vi "7L19-c-stockage_oui_non.vi"(5 "err in":errorcluster, 8 "Pénalité (e)":T2, 9 "Pièce (e)":T1) -> (1 "Stockage (sortie)":T3, 2 "Pénalité (s)":T2, 3 "Pièce (s)":T1, 4 "err out":errorcluster)   [LabVIEW 2010, in "lv_07.lvlib"]
doc: "Evalue dans la commande Stockage si la pièce peut être stockée - \n- Valeur de Qa min à comparer à Qa\n- CDM > CSM ?"
uses:
  lv_07.lvlib
  c_pi_wilson.ctl
  c_pi_penalite.ctl
  c_pi_stock.ctl
  c_pi_stock_O-N.ctl
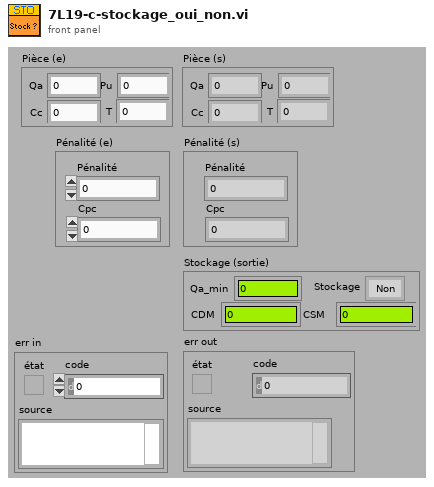
[diagram p1: front panel]
types:
  T1 = typedef "lv_07.lvlib/c_pi_wilson.ctl" = cluster{"T":dbl, "Pu":dbl, "Qa":dbl, "Cc":dbl}
  T2 = typedef "lv_07.lvlib/c_pi_penalite.ctl" = cluster{"Pénalité":dbl, "Cpc":dbl}
  T3 = typedef "lv_07.lvlib/c_pi_stock.ctl" = cluster{"Qa_min":dbl, "CDM":dbl, "CSM":dbl, "Stockage":T4}
  T4 = typedef "lv_07.lvlib/c_pi_stock_O-N.ctl" = enum16{"Non", "Oui"}
  T5 = typedef "lv_07.lvlib/c_cout_choix_q.ctl" = cluster{"Cadm":dbl, "Cpos":dbl, "Cach":dbl, "CSM":dbl, "q":dbl, "T en mois":dbl}
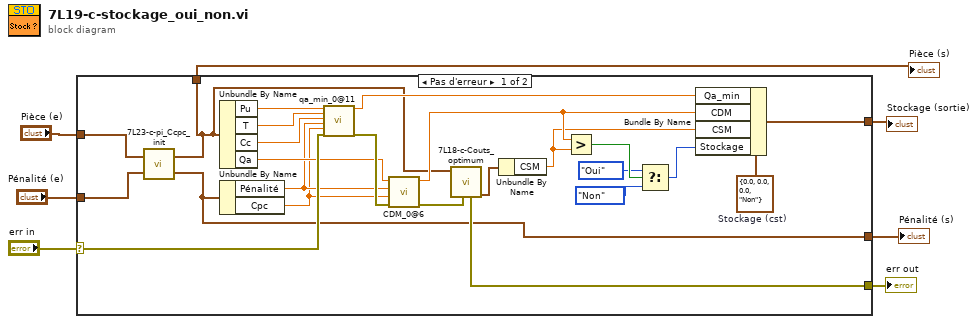
[diagram p0: block diagram]
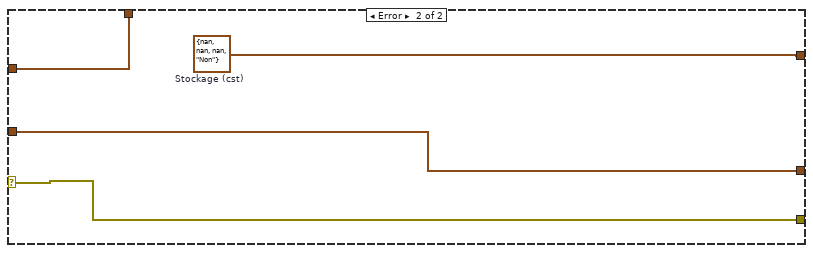
[diagram p2: hidden frame]
diagram:
  n1 = case shown="Pas d'erreur" "err in" {
    selector: "err in" -> [w30 w35]
    tunnel: [w17 w35] -> w6
    tunnel: [w16 w34] -> w5
    tunnel: "Pénalité (e)" -> [w11 w33]
    tunnel: "Pièce (e)" -> [w10 w32]
    tunnel: [w8 w33] -> w2
    tunnel: [w9 w32] -> w1
    frame No Error {
      w31 = T3 {"Qa_min"=0.0, "CDM"=0.0, "CSM"=0.0, "Stockage"=enum."Non"}  # Stockage (cst)
      n2 = call "7L23-c-pi_Ccpc_init.vi"("Pénalité (e)"=w11, "Pièce e"=w10) -> ("Pénalité (s)"=w8:T2, "Pièce s"=w9:T1)
      n3 = Unbundle By Name(w9) -> ("Pu"=w27:dbl, "T"=w28:dbl, "Cc"=w29:dbl, "Qa"=w24:dbl)
      n4 = Unbundle By Name(w8) -> ("Pénalité"=w23:dbl, "Cpc"=w22:dbl)
      n5 = call "qa_min_0@11.vi"("Pu"=w27, "T"=w28, "Cc"=w29, "Pénalité"=w23, "Cpc"=w22, "error in (no error)"=w30) -> ("Qa min"=w26:dbl, "error out"=w25:errorcluster)  [unwired: 12 in]
      n6 = call "CDM_0@6.vi"("err in"=w25, "Cpc"=w22, "Pénalité"=w23, "Qa"=w24) -> ("err out"=w21:errorcluster, "CDM"=w19:dbl)  [unwired: 6 in]
      n7 = call "7L18-c-Couts_optimum.vi"("error in"=w21, "Pièce"=w9) -> ("Coût (q=Qe)"=w20:T5, "error out"=w17:errorcluster)  [unwired: 5 in, 1 out]
      n8 = Unbundle By Name(w20) -> ("CSM"=w18:dbl)
      n9 = Greater?(x=w19, y=w18) -> (0:w15:bool)
      n10 = Select(t=c_pi_stock_O-N."Oui" ("Stockage"), s=w15, f=c_pi_stock_O-N."Non" ("Stockage")) -> (s? t:f=w14:T4)
      n11 = Bundle By Name(cluster=w31, "Qa_min"=w26, "CDM"=w19, "CSM"=w18, "Stockage"=w14) -> (w16:T3)
    }
    frame Error {
      w34 = T3 {"Qa_min"=nan, "CDM"=nan, "CSM"=nan, "Stockage"=enum."Non"}  # Stockage (cst)
    }
  }
  "err out" <- w6
  "Stockage (sortie)" <- w5
  "Pénalité (s)" <- w2
  "Pièce (s)" <- w1
